vi "VisitLVEnumType.vi"(8 "error in (no error)":errorcluster, 10 "LVEnumType":refnum<class "LVEnum.lvclass">, 11 "NextGenXMLTypeGenerator in":refnum<class "NextGenXMLTypeGenerator.lvclass">) -> (0 "error out":errorcluster, 3 "NextGenXMLTypeGenerator out":refnum<class "NextGenXMLTypeGenerator.lvclass">)   [LabVIEW 2020, in "Web Service Description.lvlib" / "NextGenXMLTypeGenerator.lvclass"]
uses:
  <vilib>/AppBuilder/Engine/WebServiceDescription/NextGenXMLTypeGenerator/NextGenXMLTypeGenerator.lvclass
  <vilib>/AppBuilder/Engine/WebServiceDescription/LVDataTypes/LVEnum/LVEnum.lvclass
  <vilib>/AppBuilder/Engine/WebServiceDescription/NextGenXMLTypeGenerator/NextGenXMLTypeGenerator.lvclass/NextGenXMLTypeGenerator.ctl
  <vilib>/AppBuilder/Engine/WebServiceDescription/GetTypeAttributesVisitor/GetTypeAttributesVisitor.lvclass
  e:/builds/penguin/labview/branches/2020/dev/dist/vi.lib/AppBuilder/Engine/WebServiceDescription/LVDataTypes/LVTypeVisitor/LVTypeVisitor.lvclass
  <vilib>/AppBuilder/Engine/WebServiceDescription/XMLGen/XMLGen.lvlib
  <vilib>/AppBuilder/Engine/WebServiceDescription/Web Service Description.lvlib
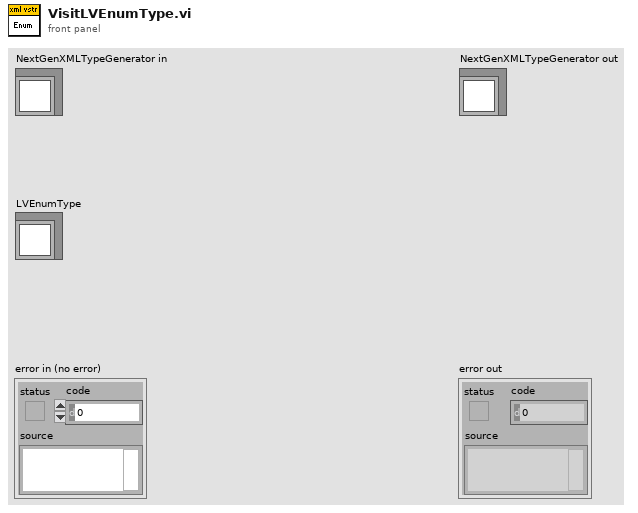
[diagram p1: front panel]
types:
  T1 = typedef "XMLGen.lvlib/ValuePair.ctl" = cluster{"Name":string, "Value":string}
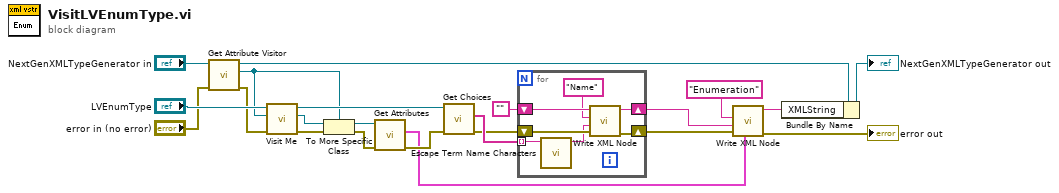
[diagram p0: block diagram]
diagram:
  n1 = call <vilib>:"Get Attribute Visitor.vi"("error in (no error)"="error in (no error)", "NextGenXMLTypeGenerator in"="NextGenXMLTypeGenerator in") -> ("error out"=w4:errorcluster, "Attribute Visitor"=w5:refnum<class "GetTypeAttributesVisitor.lvclass">, "NextGenXMLTypeGenerator out"=w3:refnum<class "NextGenXMLTypeGenerator.lvclass">)  [unwired: 7 out]
  n2 = call-dynamic "Visit Me.vi"("error in (no error)"=w4, "Visitor In"=w5, "LVEnum in"="LVEnumType") -> ("error out"=w12:errorcluster, "Visitor Out"=w11:refnum<class "LVTypeVisitor.lvclass">, "LVEnum out"=w8:refnum<class "LVEnum.lvclass">)  [unwired: 6 out]
  n3 = To More Specific Class(target class=w5, reference=w11, error in=w12) -> (specific class reference=w14:refnum<class "GetTypeAttributesVisitor.lvclass">, error out=w13:errorcluster)
  n4 = call <vilib>:"Get Attributes.vi"("error in (no error)"=w13, "GetTypeAttributesVisitor.lvclass in"=w14) -> ("error out"=w9:errorcluster, "Attributes"=w1:T1[])  [unwired: 8 out]
  n5 = call <vilib>:"Get Choices.vi"("error in (no error)"=w9, "LVEnum.lvclass in"=w8) -> ("error out"=w2:errorcluster, "Choices"=w21:string[])  [unwired: 8 out]
  n6 = for {
    shift-right: [w25] -> w18
    shift-left: "" -> [w29]
    shift-right: [w26] -> w20
    shift-left: w2 -> [w27]
    tunnel: w21 -> [w24] mode=indexing
    n7 = call <vilib>:"Escape Term Name Characters.vi"("terminal name in"=w24) -> ("terminal name out"=w23:string)  [unwired: 10 in]
    n8 = call <vilib>:"Write XML Node.vi"("error in (no error)"=w27, "body"=w23, "node"="Name", "initial string"=w29) -> ("error out"=w26:errorcluster, "resulting string"=w25:string)  [unwired: 1 in, 5 out]
  }
  n9 = call <vilib>:"Write XML Node.vi"("attributes"=w1, "error in (no error)"=w20, "body"=w18, "node"="Enumeration") -> ("error out"=→"error out":errorcluster, "resulting string"=w16:string)  [unwired: 1 in, 5 out]
  n10 = Bundle By Name(cluster=w3, "XMLString"=w16) -> (→"NextGenXMLTypeGenerator out":refnum<class "NextGenXMLTypeGenerator.lvclass">)
